vi "LWXPS_PositionerPositionCompareGet.vi"(0 "XPS Reference IN":refnum<k24>, 2 "Positioner Name":string, 5 "LabVIEW error IN":errorcluster) -> (12 "XPS Reference OUT":refnum<k24>, 13 "LabVIEW error OUT":errorcluster, 14 "Returned error code":i32, 15 "Minimum position":dbl, 16 "Maximum position":dbl, 17 "Position step":dbl, 18 "Position compare state":bool, 19 "XPS Error String":string)   [LabVIEW 2014]
uses:
  D:/XPSQ8_LabView_Library/Development/Source/Dll/Newport.XPS.CommandInterface.dll
  Dll/Newport.XPS.CommandInterface.dll
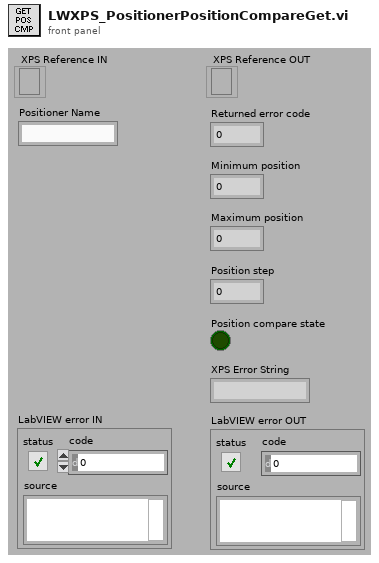
[diagram p1: front panel]
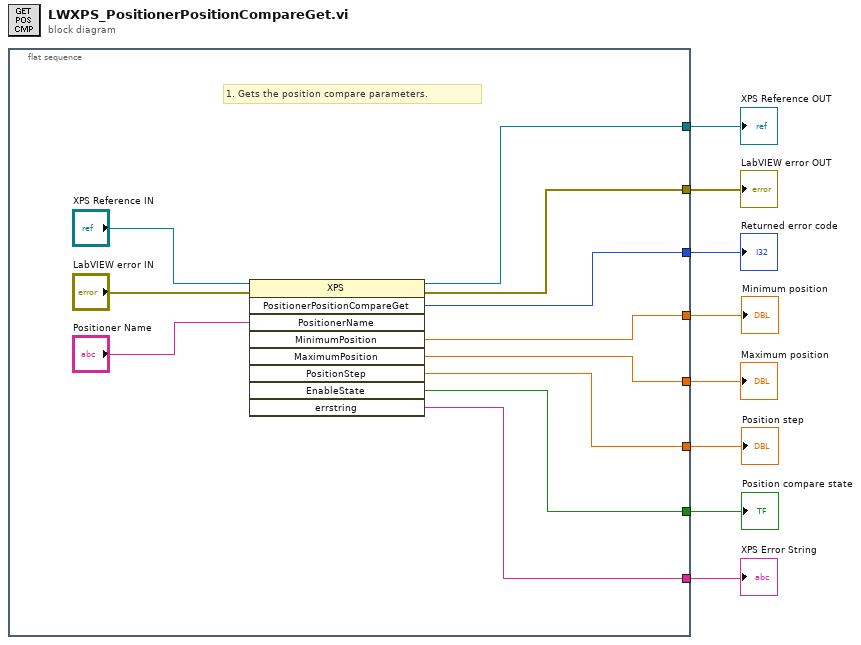
[diagram p0: block diagram]
diagram:
  n1 = flat-sequence {
    tunnel: [w17] -> w8
    tunnel: [w15] -> w7
    tunnel: [w18] -> w6
    tunnel: [w10] -> w3
    tunnel: [w14] -> w5
    tunnel: [w13] -> w2
    tunnel: [w12] -> w1
    tunnel: [w11] -> w4
    frame #0 {
      # "1. Gets the position compare parameters."
      n2 = invoke class="XPS" method="PositionerPositionCompareGet"(reference="XPS Reference IN", error in="LabVIEW error IN", "PositionerName"="Positioner Name") -> (reference out=w17:refnum<k24>, error out=w15:errorcluster, "PositionerPositionCompareGet"=w18:i32, "MinimumPosition"=w10:dbl, "MaximumPosition"=w14:dbl, "PositionStep"=w13:dbl, "EnableState"=w12:bool, "errstring"=w11:string)  [unwired: 6 in, 1 out]
    }
  }
  "XPS Error String" <- w4
  "XPS Reference OUT" <- w8
  "LabVIEW error OUT" <- w7
  "Returned error code" <- w6
  "Maximum position" <- w5
  "Minimum position" <- w3
  "Position step" <- w2
  "Position compare state" <- w1
